vi "Configure Measurement.vi"(6 "Manual Range (1)":dbl=1.0, 7 "Absolute Resolution (1E-6)":dbl=1e-06, 8 "error in (no error)":errorcluster, 9 "Auto Range (T: Enable)":bool=TRUE, 10 "Measurement Function (10: Voltage DC)":i32(ring)=10 items=["Continuity", "Current AC", "Current DC", "Diode", "Frequency", "Resistance 4-wire", "Period", "Resistance 2-wire", "Temperature", "Voltage AC", "Voltage DC", "Voltage DC Ratio"], 11 "VISA resource name":refnum<visa-resource-name>) -> (0 "error out":errorcluster, 3 "VISA resource name out":refnum<visa-resource-name>)   [LabVIEW 2014, in "Agilent 3446X Series.lvlib"]
doc: "Configures the measurement type, resolution, and range on the instrument."
uses:
  Agilent 3446X Series.lvlib
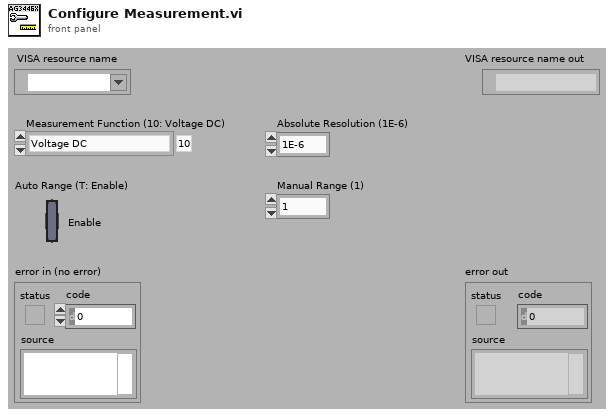
[diagram p1: front panel]
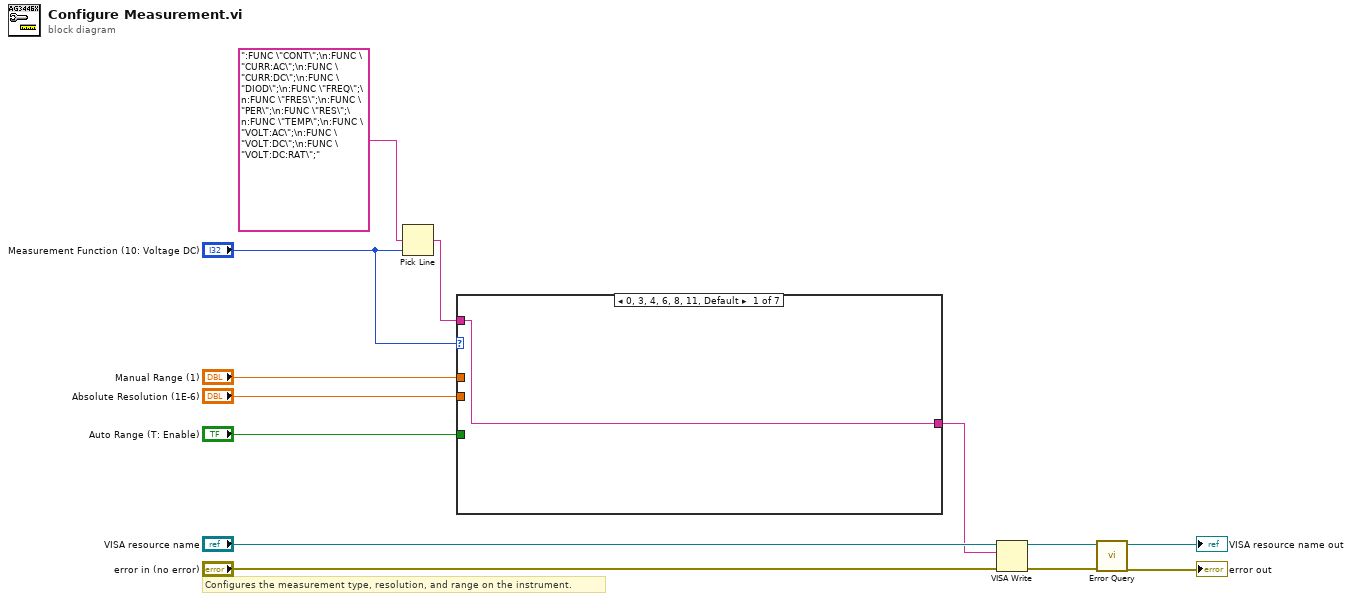
[diagram p0: block diagram]
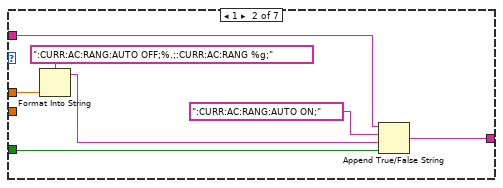
[diagram p2: hidden frame]
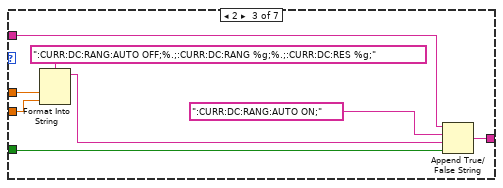
[diagram p3: hidden frame]
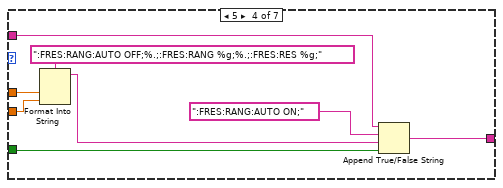
[diagram p4: hidden frame]
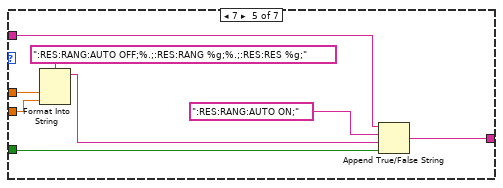
[diagram p5: hidden frame]
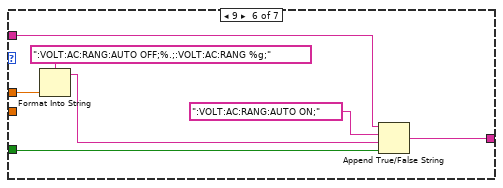
[diagram p6: hidden frame]
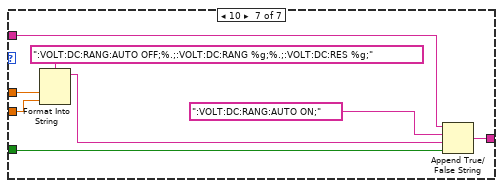
[diagram p7: hidden frame]
diagram:
  # "Configures the measurement type, resolution, and range on the instrument."
  n1 = Pick Line(multi-line string=":FUNC \"CONT\";\n:FUNC \"CURR:AC\";\n:FUNC \"CURR:DC\";\n:FUNC \"DIOD\";\n:FUNC \"FREQ\";\n:FUNC \"FRES\";\n:FUNC \"PER\";\n:FUNC \"RES\";\n:FUNC \"TEMP\";\n:FUNC \"VOLT:AC\";\n:FUNC \"VOLT:DC\";\n:FUNC \"VOLT:DC:RAT\";", line index="Measurement Function (10: Voltage DC)") -> (output string=w3:string)  [unwired: 1 out]
  n2 = case shown="0, 3, 4, 6, 8, 11, Default" "Measurement Function (10: Voltage DC)" {
    tunnel: "Manual Range (1)" -> [_ w20 w28 w36 w44 w51 w59]
    tunnel: "Auto Range (T: Enable)" -> [_ w17 w25 w33 w41 w48 w55]
    tunnel: w3 -> [w14 w16 w24 w32 w40 w47 w56]
    tunnel: [w14 w15 w22 w30 w39 w46 w53] -> w1
    tunnel: "Absolute Resolution (1E-6)" -> [_ _ w23 w31 w38 _ w54]
    frame 0, 3, 4, 6, 8, 11, Default {
    }
    frame 1 {
      n3 = Format Into String(format string=":CURR:AC:RANG:AUTO OFF;%.;:CURR:AC:RANG %g;", w20) -> (resulting string=w18:string)  [unwired: 2 in, 1 out]
      n4 = Append True/False String(1:w17, 2:w18, 3:":CURR:AC:RANG:AUTO ON;", 4:w16) -> (0:w15:string)
    }
    frame 2 {
      n5 = Format Into String(format string=":CURR:DC:RANG:AUTO OFF;%.;:CURR:DC:RANG %g;%.;:CURR:DC:RES %g;", w28, w23) -> (resulting string=w26:string)  [unwired: 2 in, 1 out]
      n6 = Append True/False String(1:w25, 2:w26, 3:":CURR:DC:RANG:AUTO ON;", 4:w24) -> (0:w22:string)
    }
    frame 5 {
      n7 = Format Into String(format string=":FRES:RANG:AUTO OFF;%.;:FRES:RANG %g;%.;:FRES:RES %g;", w36, w31) -> (resulting string=w34:string)  [unwired: 2 in, 1 out]
      n8 = Append True/False String(1:w33, 2:w34, 3:":FRES:RANG:AUTO ON;", 4:w32) -> (0:w30:string)
    }
    frame 7 {
      n9 = Format Into String(format string=":RES:RANG:AUTO OFF;%.;:RES:RANG %g;%.;:RES:RES %g;", w44, w38) -> (resulting string=w42:string)  [unwired: 2 in, 1 out]
      n10 = Append True/False String(1:w41, 2:w42, 3:":RES:RANG:AUTO ON;", 4:w40) -> (0:w39:string)
    }
    frame 9 {
      n11 = Format Into String(format string=":VOLT:AC:RANG:AUTO OFF;%.;:VOLT:AC:RANG %g;", w51) -> (resulting string=w49:string)  [unwired: 2 in, 1 out]
      n12 = Append True/False String(1:w48, 2:w49, 3:":VOLT:AC:RANG:AUTO ON;", 4:w47) -> (0:w46:string)
    }
    frame 10 {
      n13 = Format Into String(format string=":VOLT:DC:RANG:AUTO OFF;%.;:VOLT:DC:RANG %g;%.;:VOLT:DC:RES %g;", w59, w54) -> (resulting string=w57:string)  [unwired: 2 in, 1 out]
      n14 = Append True/False String(1:w55, 2:w57, 3:":VOLT:DC:RANG:AUTO ON;", 4:w56) -> (0:w53:string)
    }
  }
  n15 = VISA Write(VISA resource name="VISA resource name", write buffer=w1, error in (no error)="error in (no error)") -> (VISA resource name out=w10:refnum<visa-resource-name>, error out=w9:errorcluster)  [unwired: 1 out]
  n16 = call "Error Query.vi"("error in (no error)"=w9, "VISA resource name"=w10) -> ("error out"=→"error out":errorcluster, "VISA resource name out"=→"VISA resource name out":refnum<visa-resource-name>)  [unwired: 8 out]
